vi "Generate INSERT Query for Transaction Table.vi"(8 "error in (no error)":errorcluster, 11 "Banking Statement in":refnum<class "Banking Transactions.lvclass">) -> (0 "error out":errorcluster, 2 "Insert Query":string, 3 "Banking Statement out":refnum<class "Banking Transactions.lvclass">)   [LabVIEW 2018, in "Banking Transactions.lvclass"]
uses:
  Banking Transactions.lvclass
  Statement/TransactionList.lvclass
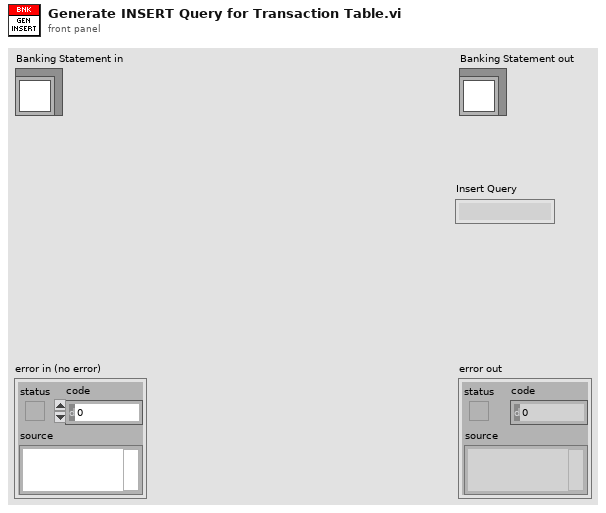
[diagram p1: front panel]
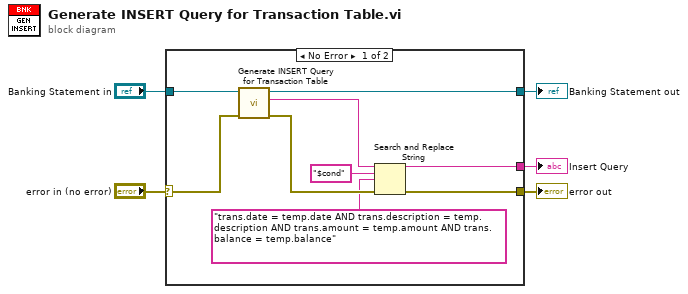
[diagram p0: block diagram]
diagram:
  n1 = case shown="No Error" "error in (no error)" {
    selector: "error in (no error)" -> [w6 w15]
    tunnel: [w14 w16] -> w5
    tunnel: "Banking Statement in" -> [w13 w16]
    tunnel: [w11 w15] -> w3
    tunnel: [w8 _] -> w2
    frame No Error {
      n2 = call-parent "Generate INSERT Query for Transaction Table.vi"("error in (no error)"=w6, "Statement in"=w13) -> ("error out"=w12:errorcluster, "Insert Query"=w10:string, "Statement out"=w14:refnum<class "Banking Transactions.lvclass">)  [unwired: 7 in]
      n3 = Search and Replace String(input string=w10, search string="$cond", replace string="trans.date = temp.date AND trans.description = temp.description AND trans.amount = temp.amount AND trans.balance = temp.balance", error in=w12) -> (result string=w8:string, error out=w11:errorcluster)  [unwired: 4 in, 2 out]
    }
    frame Error {
    }
  }
  "error out" <- w3
  "Banking Statement out" <- w5
  "Insert Query" <- w2
